vi "Stock Design Exists.vi"(8 "error in (no error)":errorcluster, 9 "Request File Name":string, 10 "Revision":i32, 11 "Method":string) -> (0 "error out":errorcluster, 3 "file or folder exists?":bool)   [LabVIEW 2012]
uses:
  Folders.ctl
  Design Server.lvlib
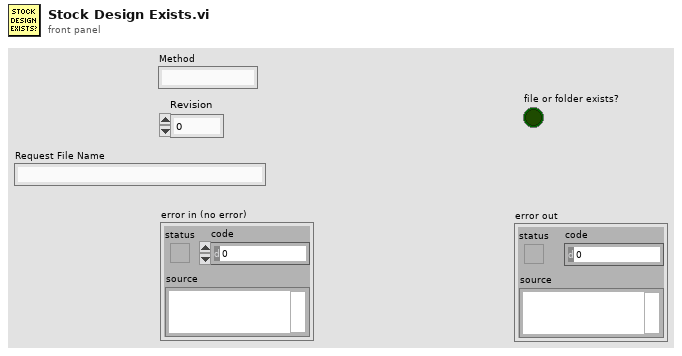
[diagram p1: front panel]
types:
  T1 = typedef "Design Server.lvlib/Folders.ctl" = enum16{"MathcadMethods", "RequestedDesigns", "CompletedDesigns", "MathcadCode", "CollabnetSVN.exe"}
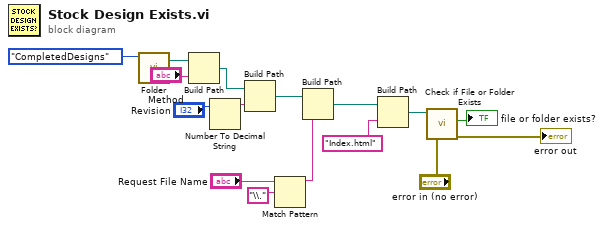
[diagram p0: block diagram]
diagram:
  n1 = call "Folder.vi"("Folders"=Folders."CompletedDesigns") -> ("FolderPath"=w15:path)  [unwired: 8 in, 2 out]
  n2 = Build Path(base path=w15, name or relative path="Method") -> (appended path=w8:path)
  n3 = Number To Decimal String(number="Revision") -> (decimal integer string=w13:string)  [unwired: 1 in]
  n4 = Build Path(base path=w8, name or relative path=w13) -> (appended path=w7:path)
  n5 = Match Pattern(string="Request File Name", regular expression="\\.") -> (before substring=w9:string)  [unwired: 1 in, 3 out]
  n6 = Build Path(base path=w7, name or relative path=w9) -> (appended path=w3:path)
  n7 = Build Path(base path=w3, name or relative path="Index.html") -> (appended path=w2:path)
  n8 = call <vilib>:"Check if File or Folder Exists.vi"("error in (no error)"="error in (no error)", "path"=w2) -> ("error out"=→"error out":errorcluster, "file or folder exists?"=→"file or folder exists?":bool)  [unwired: 7 in, 1 out]
